vi "v2sUmrechnung.vi"(0 "Impact Speed [m/s]":dbl, 1 "Test Subject h":dbl) -> (4 "Hight":dbl, 6 "?":bool)   [LabVIEW 2020]
panel:
  in  "Reibung [m/s^2]":dbl
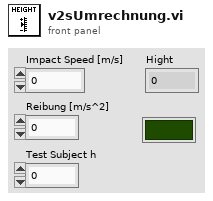
[diagram p1: front panel]
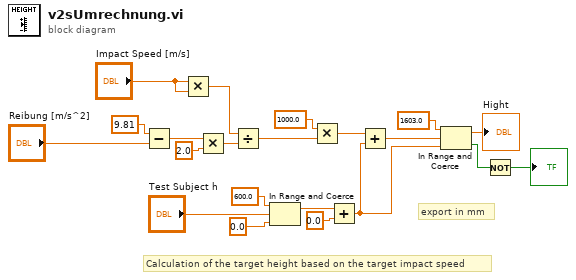
[diagram p0: block diagram]
diagram:
  # "export in mm"
  # "Calculation of the target height based on the target impact speed"
  n1 = Subtract(x=9.81 ("Zielposition"), y="Reibung [m/s^2]") -> (x-y=w15:dbl)
  n2 = Multiply(x="Impact Speed [m/s]", y="Impact Speed [m/s]") -> (x*y=w20:dbl)
  n3 = Multiply(x=w15, y=2.0 ("Zielposition")) -> (x*y=w21:dbl)
  n4 = Divide(x=w20, y=w21) -> (x/y=w3:dbl)
  n5 = In Range and Coerce(upper limit=600.0 ("Obergrenze"), x="Test Subject h", lower limit=0.0 ("Untergrenze")) -> (coerced(x)=w9:dbl)  [unwired: 1 out]
  n6 = Multiply(x=1000.0, y=w3) -> (x*y=w2:dbl)
  n7 = Add(x=w9, y=0.0 ("Wert")) -> (x+y=w7:dbl)
  n8 = Add(x=w2, y=w7) -> (x+y=w8:dbl)
  n9 = In Range and Coerce(upper limit=1603.0 ("Obergrenze"), x=w8, lower limit=w7) -> (coerced(x)=→"Hight":dbl, In Range?=w6:bool)
  n10 = Not(x=w6) -> (.not. x?=→"?":bool)
